vi "Example Read MXRPM.vi"() -> ()   [LabVIEW 2017]
uses:
  <instrlib>/Roboteq Controller KBL1xxx/Roboteq Controller KBL1xxx.lvlib
panel:
  out "MXRPM":dbl format="%#_13g"
  out "Receive Answer":string
  out "Sent Command":string
  in  "Controller VISA resource name":refnum<visa-resource-name>
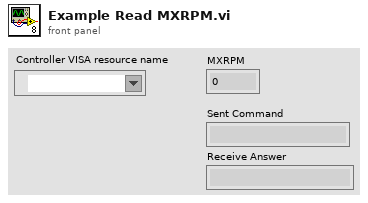
[diagram p1: front panel]
types:
  T1 = typedef "Roboteq Controller KBL1xxx.lvlib/Controller.ctl" = cluster{"VISA resource name out":refnum<visa-resource-name>, "MXRPM":u16}
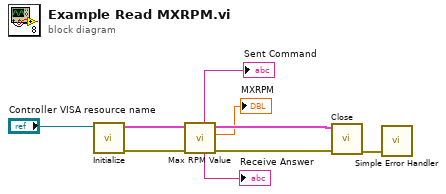
[diagram p0: block diagram]
diagram:
  n1 = call <instrlib>:"Initialize.vi"("VISA resource name"="Controller VISA resource name") -> ("error out"=w8:errorcluster, "Controller"=w7:T1)  [unwired: 9 in]
  n2 = call <instrlib>:"Max RPM Value.vi"("error in (no error)"=w8, "Controller in"=w7) -> ("error out"=w5:errorcluster, "MXRPM"=→"MXRPM":dbl, "Controller out"=w6:T1, "Receive Answer"=→"Receive Answer":string, "Sent Command"=→"Sent Command":string)  [unwired: 5 in]
  n3 = call <instrlib>:"Close.vi"("error in (no error)"=w5, "Controller in"=w6) -> ("error out"=w4:errorcluster)  [unwired: 9 in]
  n4 = call <vilib>:"Simple Error Handler.vi"("error in (no error)"=w4) -> ()  [unwired: 4 in, 5 out]
